vi "Insert Rows At (Variant).vi"(8 "error in (no error)":errorcluster, 9 "Data":variant[][](array[variant]), 10 "index":i32, 11 "DataTable in":refnum<class "DataTable.lvclass">) -> (0 "error out":errorcluster, 3 "DataTable out":refnum<class "DataTable.lvclass">)   [LabVIEW 2016, in "DataGrid.lvlib" / "DataTable.lvclass"]
doc: "This allows any number of rows to be added to the datatable. The data must match the columns defined for the grid."
uses:
  <userlib>/LabVIEWdotNetDataGrid/source/DataTable/DataTable.lvclass
  <userlib>/LabVIEWdotNetDataGrid/source/DataTable/DataTable.lvclass/DataTable.ctl
  System.Data
  <userlib>/LabVIEWdotNetDataGrid/source/GridColumn/GridColumn.lvclass/GridColumn.ctl
  <userlib>/LabVIEWdotNetDataGrid/source/GridColumn/Read datatype.vi
  <userlib>/LabVIEWdotNetDataGrid/source/GridColumn/GridColumn.lvclass
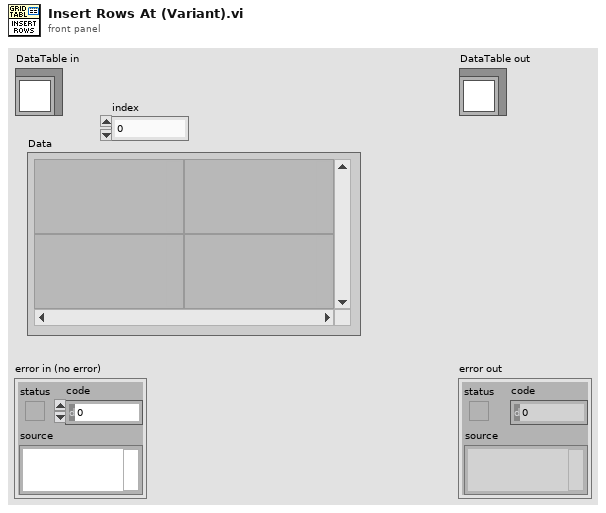
[diagram p1: front panel]
types:
  T1 = typedef "DataGrid.lvlib/GridColumn.lvclass/ColumnType.ctl" = enum16{"string", "image", "check", "numeric", "timestamp", "button", "combo", "link"}
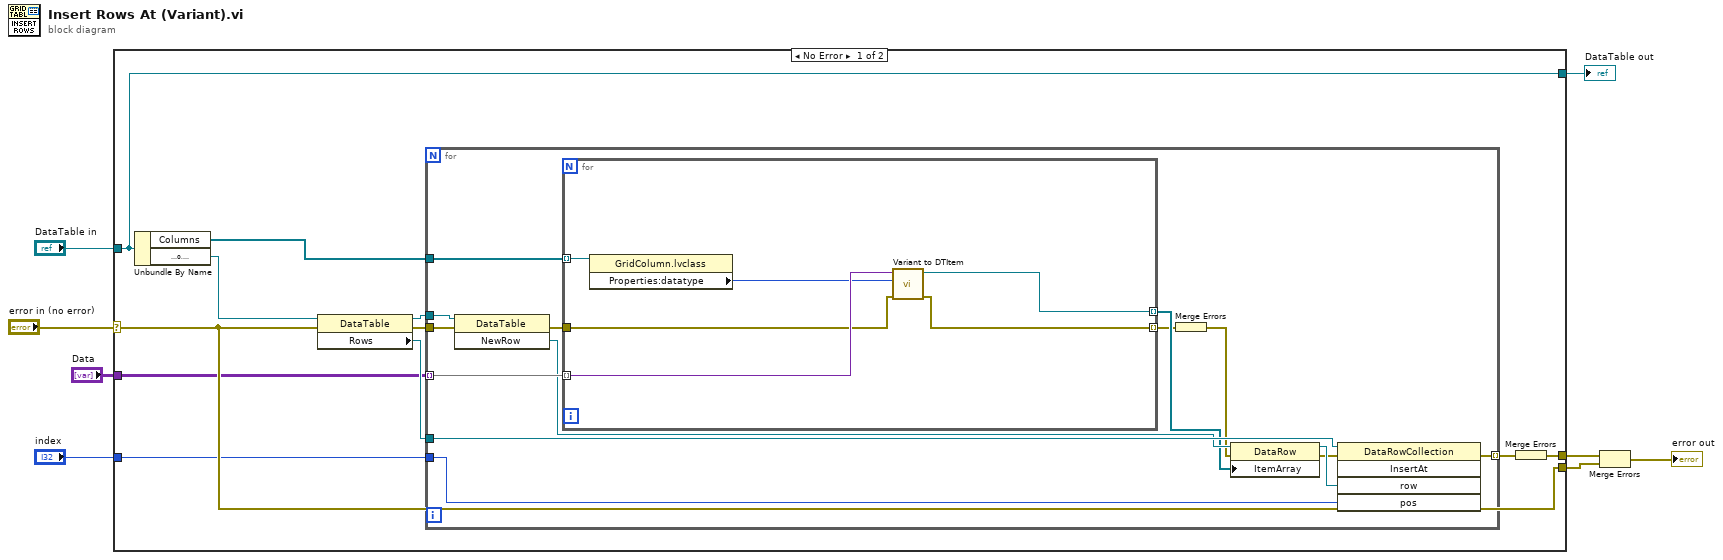
[diagram p0: block diagram]
diagram:
  n1 = case shown="No Error" "error in (no error)" {
    selector: "error in (no error)" -> [w15 w41]
    tunnel: [w15 w41] -> w7
    tunnel: [w16 w40] -> w5
    tunnel: "DataTable in" -> [w16 w40]
    tunnel: "Data" -> [w14 _]
    tunnel: [w12 _] -> w2
    tunnel: "index" -> [w9 _]
    frame No Error {
      n2 = Unbundle By Name(w16) -> ("Columns"=w11:refnum<class "GridColumn.lvclass">[], "DataTable"=w10:refnum<k24>)
      n3 = property class="DataTable"(reference=w10, error in=w15) -> (reference out=w13:refnum<k24>, error out=w19:errorcluster, "Rows"=w18:refnum<k24>)
      n4 = for {
        tunnel: w18 -> [w32]
        tunnel: w13 -> [w33]
        tunnel: [w31] -> w17 mode=indexing
        tunnel: w14 -> [w30] mode=indexing
        tunnel: w19 -> [w22]
        tunnel: w11 -> [w21]
        tunnel: w9 -> [w20]
        n5 = invoke class="DataTable" method="NewRow"(reference=w33, error in=w22) -> (error out=w29:errorcluster, "NewRow"=w28:refnum<k24>)  [unwired: 1 in, 1 out]
        n6 = for {
          tunnel: w30 -> [w38] mode=indexing
          tunnel: [w34] -> w26 mode=indexing
          tunnel: w29 -> [w36]
          tunnel: [w35] -> w25 mode=indexing
          tunnel: w21 -> [w39] mode=indexing
          n7 = property class="GridColumn.lvclass"(reference=w39) -> ("Properties:datatype"=w37:T1)  [unwired: 1 in, 2 out]
          n8 = call <userlib>:"Variant to DTItem.vi"("error in (no error)"=w36, "datatype"=w37, "element"=w38) -> ("error out"=w35:errorcluster, "DTItem .NET Refnum out"=w34:refnum<k24>)  [unwired: 7 in]
        }
        n9 = Merge Errors(w25) -> (w24:errorcluster)
        n10 = property class="DataRow"(reference=w28, error in=w24, "ItemArray"=w26) -> (reference out=w27:refnum<k24>, error out=w23:errorcluster)
        n11 = invoke class="DataRowCollection" method="InsertAt"(reference=w32, error in=w23, "row"=w27, "pos"=w20) -> (error out=w31:errorcluster)  [unwired: 1 in, 4 out]
      }
      n12 = Merge Errors(w17) -> (w12:errorcluster)
    }
    frame Error {
    }
  }
  "DataTable out" <- w5
  n13 = Merge Errors(w2, w7) -> (→"error out":errorcluster)
